vi "Read_Write_Template.vi"(0 "Template File":path, 1 "Mode":T1, 5 "Channel names In":string[](array[string]), 7 "Single Value In":string, 9 "2D Info In":string[][](array[string]), 11 "1D Info In":string[](array[string]), 12 "Save file":bool=TRUE, 13 "Data type":string="Tolerance") -> (3 "Freshly Loaded?":bool, 4 "Template File Out":path, 6 "Template Ch Names Out":string[](array[string]), 8 "Single Value Out":string, 10 "2D Info Out":string[][](array[string]), 14 "Template Info":string[][](array[string]), 15 "1D Info Out":string[](array[string]))   [LabVIEW 2015]
uses:
  Controls/Global_mode.ctl
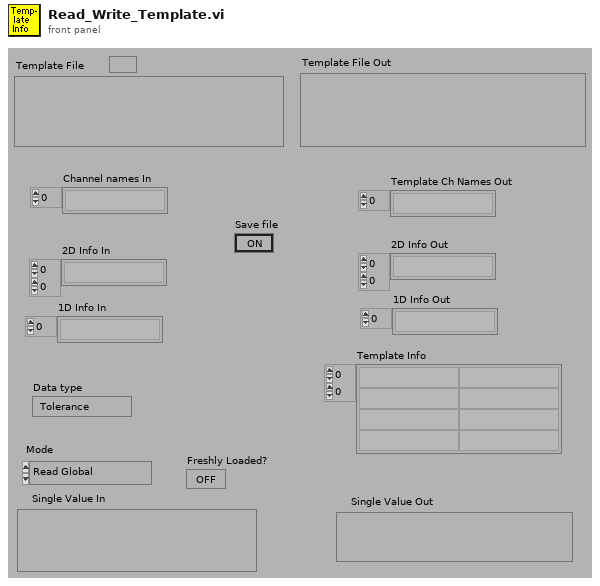
[diagram p1: front panel]
types:
  T1 = typedef "Global_mode.ctl" = enum16{"Read Global", "Load Global From File", "Write Global to File"}
  T2 = typedef "File_Status.ctl" = enum16{"Invalid Path", "This is a folder pathname", "Generic File Error", "Directory structure cannot be created", "File cannot be created", "File can be created", "File exist but read only", "File exist but no access", "File exist with read and write access"}
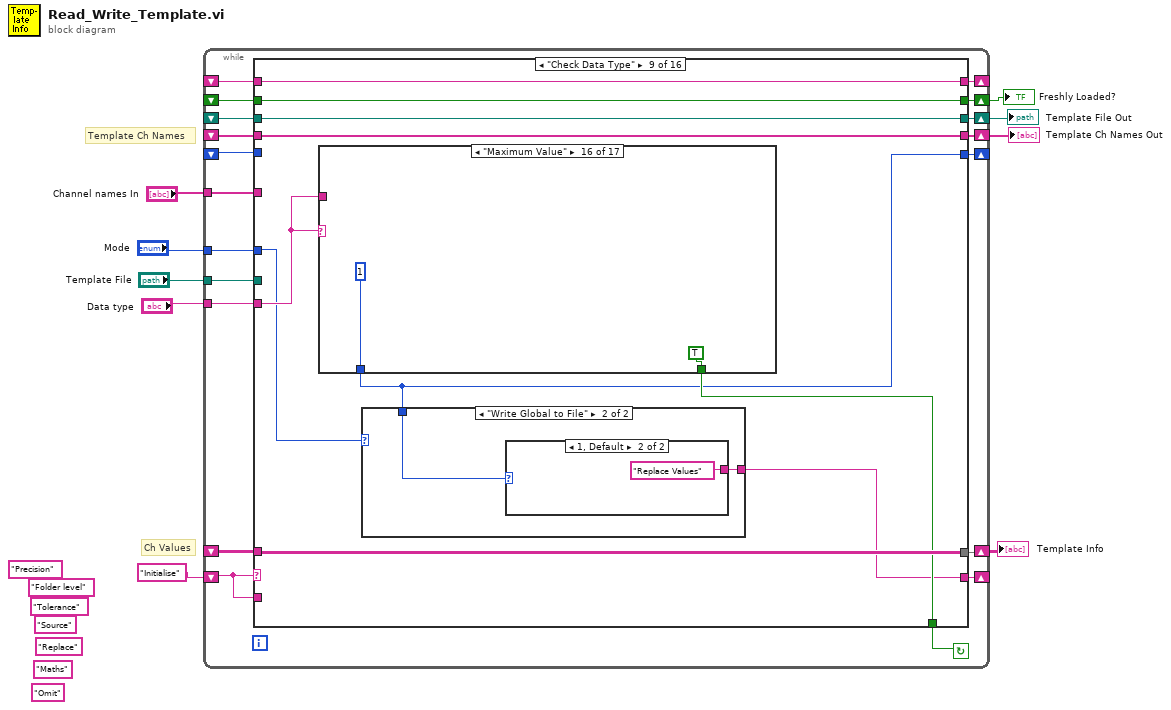
[diagram p0: block diagram]
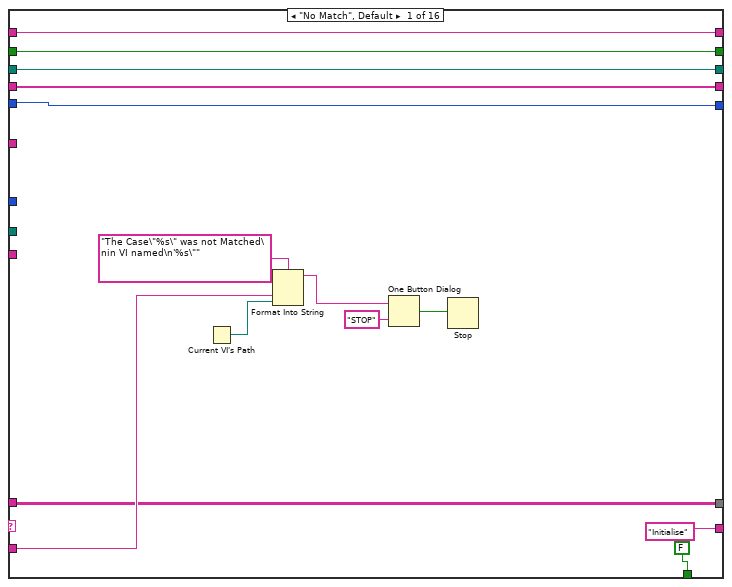
[diagram p2: hidden frame]
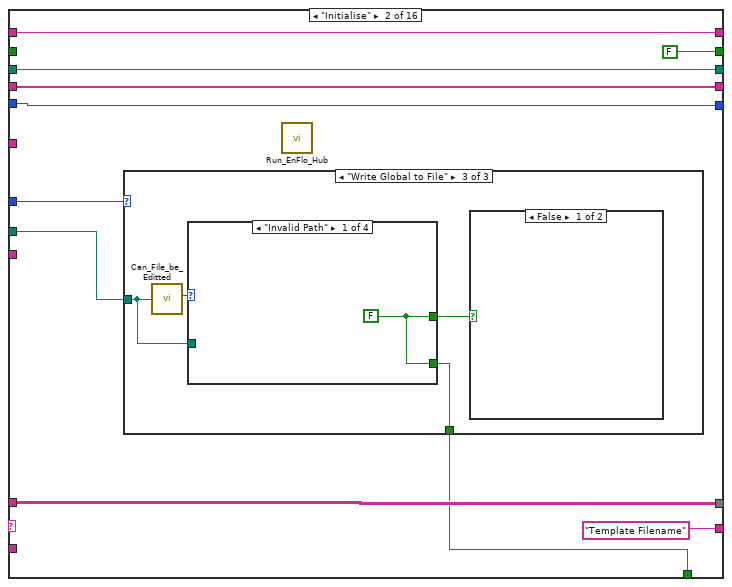
[diagram p3: hidden frame]
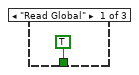
[diagram p4: hidden frame]
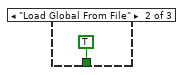
[diagram p5: hidden frame]
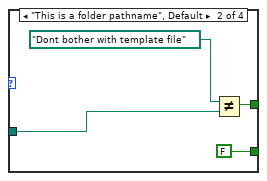
[diagram p6: hidden frame]
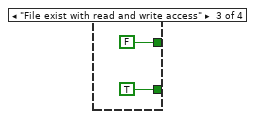
[diagram p7: hidden frame]
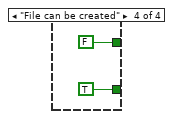
[diagram p8: hidden frame]
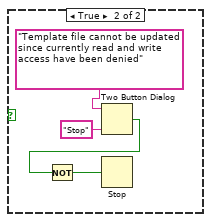
[diagram p9: hidden frame]
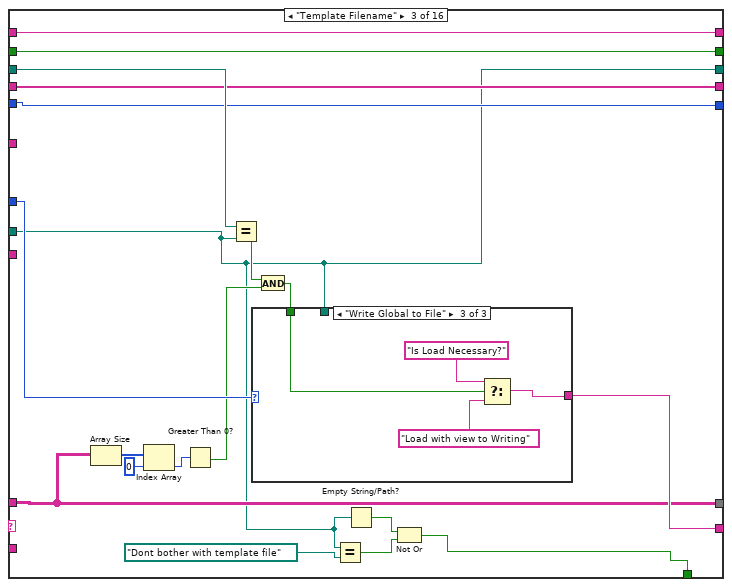
[diagram p10: hidden frame]
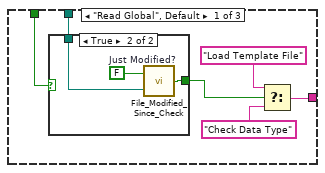
[diagram p11: hidden frame]
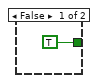
[diagram p12: hidden frame]
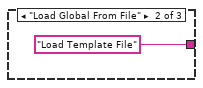
[diagram p13: hidden frame]
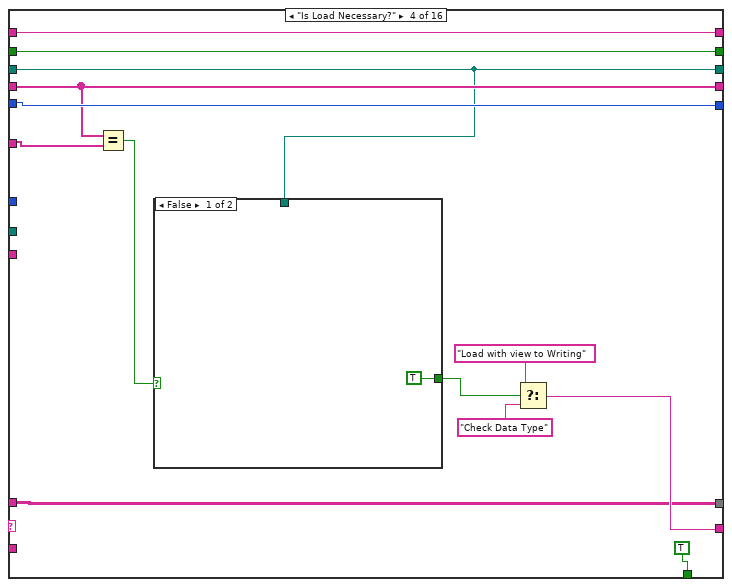
[diagram p14: hidden frame]
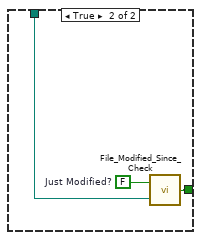
[diagram p15: hidden frame]
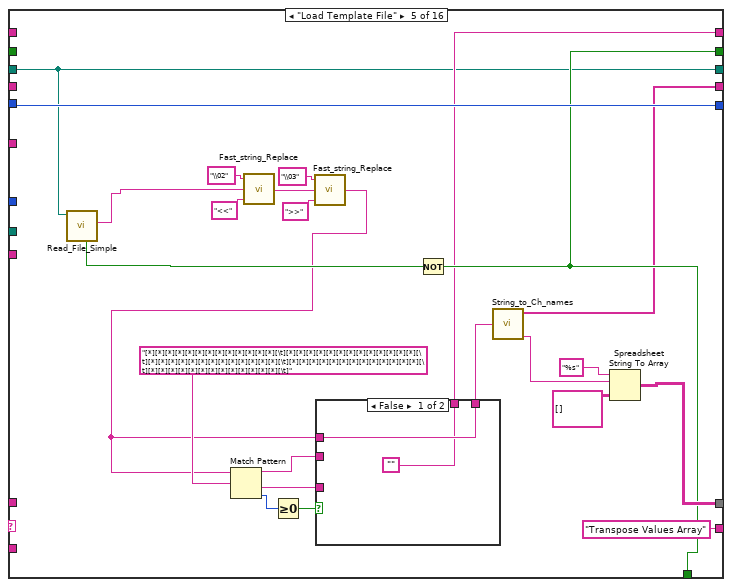
[diagram p16: hidden frame]
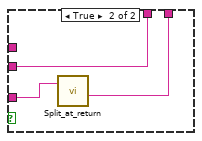
[diagram p17: hidden frame]
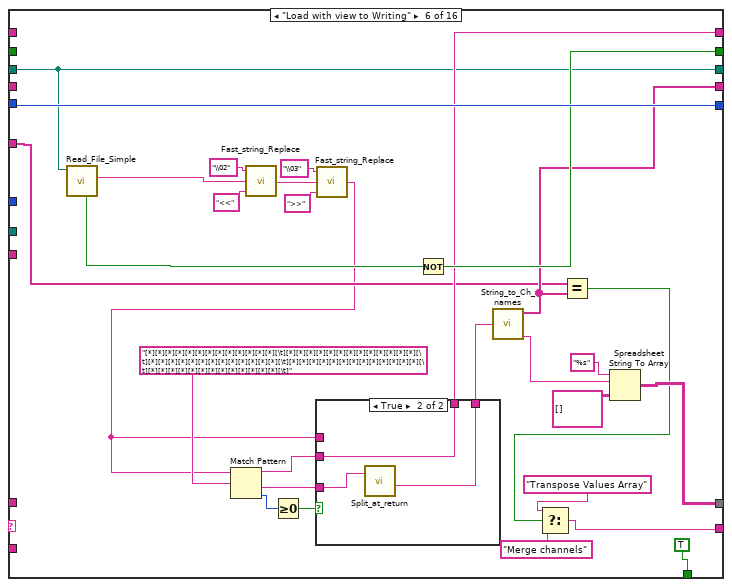
[diagram p18: hidden frame]
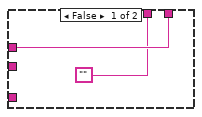
[diagram p19: hidden frame]
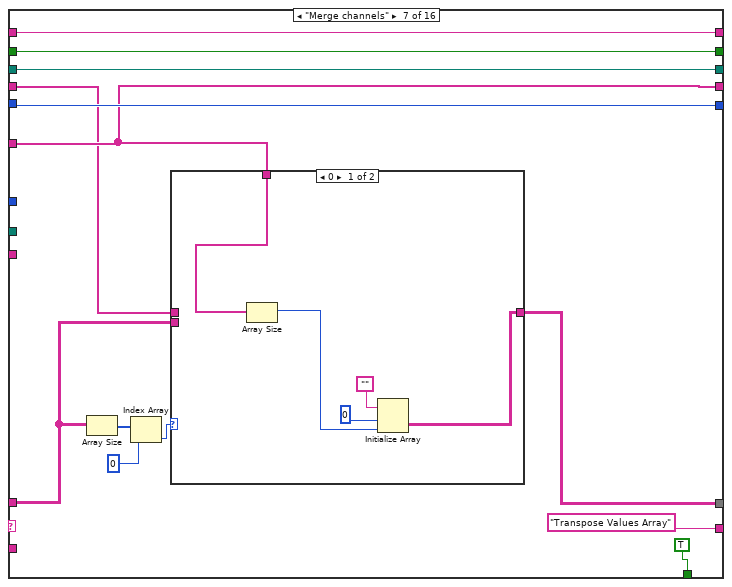
[diagram p20: hidden frame]
diagram:
  (unwired) "Precision"
  (unwired) "Folder level"
  (unwired) "Omit"
  (unwired) "Maths"
  (unwired) "Tolerance"
  (unwired) "Source"
  (unwired) "Replace"
  # "Template Ch Names"
  # "Ch Values"
  n1 = while {
    shift-left: _ -> [w13]
    shift-right: [w14] -> w2
    tunnel: "Channel names In" -> [w16]
    shift-left: _ -> [w15]
    shift-right: [w17] -> _
    tunnel: "Data type" -> [w18]
    shift-left: _ -> [w19]
    shift-right: [w20] -> w5
    shift-left: _ -> [w23]
    shift-right: [w22] -> w6
    shift-left: _ -> [w24]
    shift-right: [w25] -> w7
    tunnel: "Mode" -> [w26]
    shift-left: "Initialise" -> [w21]
    shift-right: [w27] -> _
    shift-right: [w12] -> _
    shift-left: _ -> [w11]
    tunnel: "Template File" -> [w10]
    stop <- w28 continue-if-true
    n2 = case shown="\"Check Data Type\"" w21 {
      tunnel: [FALSE w43 w73 TRUE w139 TRUE ("Save file") TRUE ("Save file") TRUE w231 FALSE FALSE FALSE "Save file" FALSE ("Save file") w461 FALSE] -> w28
      tunnel: ["Initialise" "Template Filename" w87 w118 "Transpose Values Array" w162 "Transpose Values Array" "Check Data Type" w228 "" "" "" "Save Template File" "End" w458 "End"] -> w27
      tunnel: w26 -> [_ w45 w88 _ _ _ _ _ w230 _ _ _ _ _ _ _]
      tunnel: [w33 w51 w83 w112 w143 w178 w191 w218 w234 w300 w314 w334 w360 w447 w456 w506] -> w25
      tunnel: w24 -> [w33 w51 w83 w112 _ _ w189 w217 w234 w300 w314 w334 w361 w447 w455 w506]
      tunnel: w23 -> [w35 w52 w90 w108 w131 w159 w194 w213 w233 w302 w320 w336 w362 w441 w460 w505]
      tunnel: [w35 w52 w72 w108 w131 w159 w194 w213 w233 w302 w320 w336 w362 w441 w460 w505] -> w22
      tunnel: w21 -> [w37 _ _ _ _ _ _ _ _ _ _ _ _ _ _ _]
      tunnel: [w36 w50 w89 w111 w130 w166 w193 w212 w232 w298 w315 w331 w355 w450 w459 w504] -> w20
      tunnel: w19 -> [w36 w50 w89 w111 _ _ w192 w212 w232 w298 w315 w331 w355 w450 w459 w504]
      tunnel: w18 -> [_ _ _ _ _ _ _ _ w235 w301 w312 w335 w358 w443 _ _]
      tunnel: [w31 w48 w82 w116 w145 w180 w197 w211 w229 w291 w317 w323 w353 w449 w457 w502] -> w17
      tunnel: w16 -> [_ _ _ w110 _ w165 w193 _ _ w292 _ w328 w354 _ _ _]
      tunnel: w15 -> [w31 w48 w82 w116 w145 w180 w197 w211 _ w291 w317 w323 w353 w449 w457 w502]
      tunnel: [w30 FALSE w78 w107 w139 w174 w195 w209 w227 w290 w316 w322 w352 w448 w454 w500] -> w14
      tunnel: w13 -> [w30 _ w78 w107 _ _ w195 w209 w227 w290 w316 w322 w352 w448 w454 w500]
      tunnel: [w29 w46 w77 w106 w133 w168 w196 w208 w226 w289 w313 w321 w350 w445 w452 w499] -> w12
      tunnel: w11 -> [w29 w46 w77 w106 _ _ w196 w208 w226 w289 w313 w321 w350 w444 w453 w499]
      tunnel: w10 -> [_ w44 w72 _ _ _ _ _ _ _ _ _ _ _ _ _]
      frame "No Match", Default {
        n3 = Current VI's Path() -> (path=w38:path)
        n4 = Format Into String(format string="The Case\"%s\" was not Matched\nin VI named\n'%s\"" ("Format String"), w37, w38) -> (resulting string=w41:string)  [unwired: 2 in, 1 out]
        n5 = One Button Dialog(message=w41, button name ("OK")="STOP") -> (true=w39:bool)
        n6 = Stop(stop? (T)=w39) -> ()
      }
      frame "Initialise" {
        n7 = case shown="\"Write Global to File\"" w45 {
          tunnel: w44 -> [_ _ w55]
          tunnel: [TRUE TRUE w56] -> w43
          frame "Read Global" {
          }
          frame "Load Global From File" {
          }
          frame "Write Global to File" {
            n8 = call "Can_File_be_Editted.vi"("Filename"=w55) -> ("File Status"=w58:T2)  [unwired: 3 out]
            n9 = case shown="\"Invalid Path\"" w58 {
              tunnel: [w59 w61 FALSE FALSE] -> w57
              tunnel: [w59 FALSE TRUE TRUE] -> w56
              tunnel: w55 -> [_ w60 _ _]
              frame "Invalid Path" {
                w59 = FALSE
              }
              frame "This is a folder pathname", Default {
                n10 = Not Equal?(x=path "Dont bother with template file" ("Template File"), y=w60) -> (x != y?=w61:bool)
              }
              frame "File exist with read and write access" {
              }
              frame "File can be created" {
              }
            }
            n11 = case shown="False" w57 {
              frame False {
              }
              frame True {
                n12 = Two Button Dialog(message="Template file cannot be updated since currently read and write access have been denied", 1:"Stop" ("F button name (\"Cancel\")")) -> (T button?=w69:bool)  [unwired: 1 out]
                n13 = Not(x=w69) -> (.not. x?=w68:bool)
                n14 = Stop(stop? (T)=w68) -> ()
              }
            }
          }
        }
        n15 = call "Run_EnFlo_Hub.vi"() -> ()  [unwired: 8 out]
      }
      frame "Template Filename" {
        n16 = Array Size(array=w83) -> (size(s)=w84:i32[])
        n17 = Index Array(array=w84, index=0 ("Index")) -> (element=w86:i32)
        n18 = Greater Than 0?(x=w86) -> (x > 0?=w79:bool)
        n19 = Equal?(x=w90, y=w72) -> (x = y?=w81:bool)
        n20 = And(x=w81, y=w79) -> (x .and. y?=w80:bool)
        n21 = case shown="\"Write Global to File\"" w88 {
          tunnel: w80 -> [w96 _ w105]
          tunnel: [w92 "Load Template File" w103] -> w87
          tunnel: w72 -> [w95 _ _]
          frame "Read Global", Default {
            n22 = case shown="True" w96 {
              tunnel: w95 -> [_ w100]
              tunnel: [TRUE ("Modified?") w99] -> w94
              frame False {
              }
              frame True {
                w98 = FALSE  # Just Modified?
                n23 = call "File_Modified_Since_Check.vi"("Pathname"=w100, "Just Modified?"=w98) -> ("Modified?"=w99:bool)
              }
            }
            n24 = Select(t="Load Template File", s=w94, f="Check Data Type") -> (s? t:f=w92:string)
          }
          frame "Load Global From File" {
          }
          frame "Write Global to File" {
            n25 = Select(t="Is Load Necessary?", s=w105, f="Load with view to Writing") -> (s? t:f=w103:string)
          }
        }
        n26 = Equal?(x=w72, y=path "Dont bother with template file" ("Template File")) -> (x = y?=w75:bool)
        n27 = Empty String/Path?(string/path=w72) -> (empty?=w74:bool)
        n28 = Not Or(1:w75, 2:w74) -> (0:w73:bool)
      }
      frame "Is Load Necessary?" {
        n29 = Equal?(x=w111, y=w110) -> (x = y?=w109:bool)
        n30 = case shown="False" w109 {
          tunnel: w108 -> [_ w122]
          tunnel: [TRUE ("Modified?") w121] -> w115
          frame False {
          }
          frame True {
            w120 = FALSE  # Just Modified?
            n31 = call "File_Modified_Since_Check.vi"("Pathname"=w122, "Just Modified?"=w120) -> ("Modified?"=w121:bool)
          }
        }
        n32 = Select(t="Load with view to Writing", s=w115, f="Check Data Type") -> (s? t:f=w118:string)
      }
      frame "Load Template File" {
        n33 = call "Read_File_Simple.vi"("Filename"=w131) -> ("Error?"=w144:bool, "string"=w129:string)  [unwired: 2 in, 6 out]
        n34 = call "Fast_string_Replace.vi"("Replace match with:"="<<" ("regular expression"), "Input String"=w129, "regular expression"="\\02") -> ("Output String"=w123:string)  [unwired: 2 out]
        n35 = call "Fast_string_Replace.vi"("Replace match with:"=">>" ("regular expression"), "Input String"=w123, "regular expression"="\\03") -> ("Output String"=w128:string)  [unwired: 2 out]
        n36 = Match Pattern(string=w128, regular expression="[*][*][*][*][*][*][*][*][*][*][*][*][*][\t][*][*][*][*][*][*][*][*][*][*][*][*][*][\t][*][*][*][*][*][*][*][*][*][*][*][*][*][\t][*][*][*][*][*][*][*][*][*][*][*][*][*][\t][*][*][*][*][*][*][*][*][*][*][*][*][*][\t]" ("String")) -> (before substring=w132:string, after substring=w137:string, offset past match=w136:i32)  [unwired: 2 out]
        n37 = Greater Or Equal To 0?(x=w136) -> (x >= 0?=w135:bool)
        n38 = case shown="False" w135 {
          tunnel: w137 -> [_ w151]
          tunnel: [w148 w150] -> w134
          tunnel: w128 -> [w148 _]
          tunnel: ["" w149] -> w133
          tunnel: w132 -> [_ w149]
          frame False {
          }
          frame True {
            n39 = call "Split_at_return.vi"("String"=w151) -> ("after substring"=w150:string)  [unwired: 1 in, 3 out]
          }
        }
        n40 = Not(x=w144) -> (.not. x?=w139:bool)
        n41 = call "String_to_Ch_names.vi"("Spreadsheet string"=w134) -> ("Ch names"=w130:string[], "String After names"=w140:string)  [unwired: 2 out]
        n42 = Spreadsheet String To Array(format string="%s", spreadsheet string=w140, array type (2D Dbl)=string[][] [] ("Channel Values")) -> (array=w143:string[][])  [unwired: 1 out]
      }
      frame "Load with view to Writing" {
        n43 = call "Read_File_Simple.vi"("Filename"=w159) -> ("Error?"=w179:bool, "string"=w153:string)  [unwired: 2 in, 6 out]
        n44 = call "Fast_string_Replace.vi"("Replace match with:"="<<" ("regular expression"), "Input String"=w153, "regular expression"="\\02") -> ("Output String"=w154:string)  [unwired: 2 out]
        n45 = call "Fast_string_Replace.vi"("Replace match with:"=">>" ("regular expression"), "Input String"=w154, "regular expression"="\\03") -> ("Output String"=w152:string)  [unwired: 2 out]
        n46 = Match Pattern(string=w152, regular expression="[*][*][*][*][*][*][*][*][*][*][*][*][*][\t][*][*][*][*][*][*][*][*][*][*][*][*][*][\t][*][*][*][*][*][*][*][*][*][*][*][*][*][\t][*][*][*][*][*][*][*][*][*][*][*][*][*][\t][*][*][*][*][*][*][*][*][*][*][*][*][*][\t]" ("String")) -> (before substring=w167:string, after substring=w172:string, offset past match=w171:i32)  [unwired: 2 out]
        n47 = Greater Or Equal To 0?(x=w171) -> (x >= 0?=w170:bool)
        n48 = case shown="True" w170 {
          tunnel: w172 -> [_ w185]
          tunnel: [w182 w184] -> w169
          tunnel: w152 -> [w182 _]
          tunnel: ["" w183] -> w168
          tunnel: w167 -> [_ w183]
          frame False {
          }
          frame True {
            n49 = call "Split_at_return.vi"("String"=w185) -> ("after substring"=w184:string)  [unwired: 1 in, 3 out]
          }
        }
        n50 = Not(x=w179) -> (.not. x?=w174:bool)
        n51 = call "String_to_Ch_names.vi"("Spreadsheet string"=w169) -> ("Ch names"=w166:string[], "String After names"=w175:string)  [unwired: 2 out]
        n52 = Equal?(x=w165, y=w166) -> (x = y?=w164:bool)
        n53 = Select(t="Transpose Values Array", s=w164, f="Merge channels") -> (s? t:f=w162:string)
        n54 = Spreadsheet String To Array(format string="%s", spreadsheet string=w175, array type (2D Dbl)=string[][] [] ("Channel Values")) -> (array=w178:string[][])  [unwired: 1 out]
      }
      frame "Merge channels" {
        n55 = Array Size(array=w189) -> (size(s)=w188:i32[])
        n56 = Index Array(array=w188, index=0) -> (element=w186:i32)
        n57 = case shown="0" w186 {
          tunnel: w193 -> [w200 w207]
          tunnel: w192 -> [_ w206]
          tunnel: w189 -> [_ w205]
          tunnel: [w199 w204] -> w191
          frame 0 {
            n58 = Array Size(array=w200) -> (size(s)=w201:i32)
            n59 = Initialize Array("", 0 ("Dimension Size"), w201) -> (w199:string[][])
          }
          frame 1, Default {
            n60 = call "Merge_2D_values.vi"("Values In"=w205, "Present Channels"=w206, "Desired Channels"=w207) -> ("Values Out"=w204:string[][])
          }
        }
      }
      frame "Transpose Values Array" {
        n61 = Array Size(array=w217) -> (size(s)=w215:i32[])
        n62 = Index Array(array=w215, index=1 ("Index")) -> (element=w214:i32)
        n63 = for {
          N: w214 -> [_]
          tunnel: w217 -> [w222]
          tunnel: [w223] -> w218 mode=indexing
          i -> [w221]
          n64 = Index Array(array=w222, index (col)=w221) -> (element=w220:string[])  [unwired: 1 in]
          n65 = for {
            tunnel: [w225] -> w223 mode=indexing
            tunnel: w220 -> [w224] mode=indexing
            n66 = call "Remove_Quotes.vi"("String"=w224) -> ("String Out"=w225:string)
          }
        }
      }
      frame "Check Data Type" {
        n67 = case shown="\"Maximum Value\"" w235 {
          tunnel: [1 1 1 1 1 2 1 1 2 2 2 1 2 1 1 1 0] -> w229
          tunnel: w235 -> [w246 _ _ _ _ _ _ _ _ _ _ _ _ _ _ _ _]
          tunnel: [w245 TRUE TRUE TRUE TRUE TRUE TRUE TRUE TRUE TRUE TRUE TRUE TRUE TRUE TRUE TRUE TRUE] -> w231
          frame "No Match", Default {
            n68 = Empty String/Path?(string/path=w246) -> (empty?=w247:bool)
            n69 = case shown="False" w247 {
              tunnel: w246 -> [w250 _]
              tunnel: [FALSE FALSE] -> w245
              frame False {
                n70 = Current VI's Path() -> (path=w251:path)
                n71 = Format Into String(format string="The Case\"%s\" was not Matched\nin VI named\n'%s\"" ("Format String"), w250, w251) -> (resulting string=w254:string)  [unwired: 2 in, 1 out]
                n72 = One Button Dialog(message=w254, button name ("OK")="STOP") -> (true=w252:bool)
                n73 = Stop(stop? (T)=w252) -> ()
              }
              frame True {
              }
            }
          }
          frame "Description" {
          }
          frame "Dispose" {
          }
          frame "Decimal" {
          }
          frame "Precision" {
          }
          frame "Multiple Sources" {
          }
          frame "Summarise" {
          }
          frame "Tolerance" {
          }
          frame "Source" {
          }
          frame "Replace" {
          }
          frame "Ignore When" {
          }
          frame "Maths" {
          }
          frame "Omit" {
          }
          frame "Folder level" {
          }
          frame "Minimum Value" {
          }
          frame "Maximum Value" {
          }
          frame "Log Folder Name" {
          }
        }
        n74 = case shown="\"Write Global to File\"" w230 {
          tunnel: w229 -> [w237 w241]
          tunnel: [w236 w242] -> w228
          frame "Read Global", Default {
            n75 = case shown="0" w237 {
              tunnel: ["Create Outputs 2D" "Create Outputs 1D" "Create single value output"] -> w236
              frame 2, Default {
              }
              frame 1 {
              }
              frame 0 {
              }
            }
          }
          frame "Write Global to File" {
            n76 = case shown="1, Default" w241 {
              tunnel: ["Replace single value" "Replace Values"] -> w242
              frame 0 {
              }
              frame 1, Default {
              }
            }
          }
        }
      }
      frame "Create Outputs 1D" {
        n77 = for {
          tunnel: w301 -> [w310]
          tunnel: w300 -> [w309] mode=indexing
          tunnel: [w308] -> w299 mode=indexing
          n78 = call "Get_Array_Subset.vi"("String Array In"=w309, "Subset Name"=w310) -> ("First Element"=w308:string)  [unwired: 4 out]
        }
        n79 = Array Size(array=w292) -> (size(s)=w294:i32)
        n80 = Equal To 0?(x=w294) -> (x = 0?=w293:bool)
        n81 = case shown="False" w293 {
          tunnel: w299 -> [w306 w307]
          tunnel: w292 -> [w305 _]
          tunnel: w298 -> [w304 _]
          tunnel: [w303 w307] -> w297
          frame False {
            n82 = call "Merge_row_values.vi"("Present Row values"=w306, "Present Channels"=w304, "Desired Channels"=w305) -> ("Desired Row values"=w303:string[])  [unwired: 1 out]
          }
          frame True {
          }
        }
        "1D Info Out" <- w297
      }
      frame "Create single value output" {
        n83 = call "Get_Characters_from_string.vi"("Input string"=w313, "Variable name"=w312) -> ("Value"=→"Single Value Out":string)  [unwired: 1 in, 1 out]
      }
      frame "Create Outputs 2D" {
        n84 = for {
          tunnel: w335 -> [w349]
          tunnel: w334 -> [w348] mode=indexing
          tunnel: [w347] -> w330 mode=indexing
          n85 = call "Get_Array_Subset.vi"("String Array In"=w348, "Subset Name"=w349) -> ("Array Subset Out"=w347:string[])  [unwired: 4 out]
        }
        n86 = Equal?(x=w331, y=w328) -> (x = y?=w326:bool)
        n87 = Array Size(array=w328) -> (size(s)=w327:i32)
        n88 = Equal To 0?(x=w327) -> (x = 0?=w325:bool)
        n89 = Or(x=w326, y=w325) -> (x .or. y?=w324:bool)
        n90 = case shown="False" w324 {
          tunnel: w331 -> [w340 _]
          tunnel: w328 -> [w339 _]
          tunnel: w330 -> [w338 w346]
          tunnel: [w337 w346] -> w329
          frame False {
            n91 = for {
              tunnel: w340 -> [w345]
              tunnel: w339 -> [w344] mode=indexing
              tunnel: w338 -> [w342]
              tunnel: [w341] -> w337 mode=indexing
              n92 = Search 1D Array(1D array=w345, element=w344) -> (index of element=w343:i32)  [unwired: 1 out]
              n93 = Index Array(array=w342, index (row)=w343) -> (element=w341:string[])  [unwired: 1 in]
            }
          }
          frame True {
          }
        }
        "2D Info Out" <- w329
      }
      frame "Replace Values" {
        n94 = for {
          tunnel: w358 -> [w371]
          tunnel: w361 -> [w370] mode=indexing
          tunnel: [w369] -> w360 mode=indexing
          tunnel: w355 -> [w368] mode=indexing
          tunnel: w353 -> [w367]
          tunnel: "1D Info In" -> [w366]
          tunnel: "2D Info In" -> [w365]
          tunnel: w355 -> [w364] mode=indexing
          tunnel: w354 -> [w363]
          n95 = stacked-sequence {
            seq-local: [_ w381 _ _ _] -> [_ _ _ w432 _]
            seq-local: [_ w380 _ _ _] -> [_ _ _ w433 _]
            seq-local: [_ _ w392 _ _] -> [_ _ _ w431 _]
            seq-local: [_ w379 _ _ _] -> [_ _ w388 _ _]
            seq-local: [w374 _ _ _ _] -> [_ _ w389 _ _]
            seq-local: [w372 _ _ _ _] -> [_ _ w387 _ _]
            tunnel: w371 -> [_ w386 _ w434 _]
            tunnel: w370 -> [_ w383 _ _ _]
            tunnel: [_ _ _ w424 _] -> w369
            tunnel: w368 -> [_ _ _ w425 _]
            tunnel: w367 -> [w373 _ _ _ _]
            tunnel: w366 -> [_ _ w391 _ _]
            tunnel: w365 -> [_ _ w390 _ _]
            tunnel: w364 -> [w376 _ _ _ _]
            tunnel: w363 -> [w375 _ _ _ _]
            frame #0 {
              n96 = Search 1D Array(1D array=w375, element=w376) -> (index of element=w372:i32)  [unwired: 1 out]
              n97 = case shown="0, Default" w372 {
                tunnel: [w377 0] -> w374
                tunnel: w373 -> [w377 _]
                frame 0, Default {
                }
                frame -1 {
                }
              }
            }
            frame #1 {
              n98 = call "Get_Array_Subset.vi"("String Array In"=w383, "Subset Name"=w386) -> ("index after match"=w382:i32, "Array Subset Out"=w379:string[], "Length before match"=w384:i32)  [unwired: 2 out]
              n99 = Array Subset(array=w383, index=0 ("Array Index"), length=w384) -> (w381:string[])
              n100 = Array Subset(array=w383, index=w382) -> (w380:string[])  [unwired: 1 in]
            }
            frame #2 {
              n101 = case shown="2, Default" w389 {
                tunnel: [w396 w420 w423] -> w392
                tunnel: w391 -> [_ w422 _]
                tunnel: w390 -> [w395 _ _]
                tunnel: w388 -> [_ _ w423]
                tunnel: w387 -> [w393 w419 _]
                frame 2, Default {
                  n102 = Index Array(array=w395, index (row)=w393) -> (element=w394:string[])  [unwired: 1 in]
                  n103 = while {
                    shift-left: _ -> [w397]
                    shift-right: [w398] -> _
                    tunnel: [w399] -> w396
                    tunnel: w394 -> [w401]
                    i -> [w402]
                    stop <- w400 continue-if-true
                    n104 = case shown="0, Default" w402 {
                      tunnel: w401 -> [w404 w407]
                      tunnel: [w405 FALSE] -> w400
                      tunnel: [w404 w410] -> w399
                      tunnel: [w403 w409] -> w398
                      tunnel: w397 -> [_ w409]
                      frame 0, Default {
                        n105 = Empty String/Path?(string/path=w404) -> (empty?=w403:bool[])
                        n106 = Or Array Elements(Boolean array=w403) -> (logical OR=w405:bool)
                      }
                      frame 1 {
                        n107 = for {
                          shift-right: [w413] -> w410
                          shift-left: string[] [] -> [w412]
                          tunnel: w409 -> [w414] mode=indexing
                          tunnel: w407 -> [w411] mode=indexing
                          n108 = case shown="True" w414 {
                            tunnel: [w416 w418] -> w413
                            tunnel: w412 -> [w417 w418]
                            tunnel: w411 -> [w415 _]
                            frame False {
                              n109 = Build Array (concatenate)(w417, w415) -> (w416:string[])
                            }
                            frame True {
                            }
                          }
                        }
                      }
                    }
                  }
                }
                frame 1 {
                  n110 = Index Array(array=w422, index=w419) -> (element=w421:string)
                  n111 = Build Array(w421) -> (w420:string[])
                }
                frame 0 {
                }
              }
            }
            frame #3 {
              w426 = ""
              n112 = Format Into String(format string="**%s Start**" ("Format String"), w434) -> (resulting string=w430:string)  [unwired: 2 in, 1 out]
              n113 = Format Into String(format string="**%s End**" ("Format String"), w434) -> (resulting string=w429:string)  [unwired: 2 in, 1 out]
              n114 = Build Array (concatenate)(w432, w430, w431, w429, w433) -> (w428:string[])
              n115 = call "Clean_Up_Template.vi"("Template Info In"=w428) -> ("Template Info Out"=w427:string[])
              n116 = Build Array (concatenate)(w426, w425, w426, w427) -> (w424:string[])
            }
            frame #4 {
            }
          }
        }
      }
      frame "Replace single value" {
        w438 = FALSE  # append to file? (new file:F)
        w439 = FALSE  # advisory dialog? (display:T)
        n117 = call "Read_File_Simple.vi"("Filename"=w441) -> ("string"=w442:string)  [unwired: 2 in, 7 out]
        n118 = call "Replace_data_in_setup_string.vi"("New data string"="Single Value In", "Input string"=w444, "Variable name"=w443) -> ("Appended string"=w445:string)
        n119 = call "Replace_data_in_setup_string.vi"("New data string"="Single Value In", "Input string"=w442, "Variable name"=w443) -> ("Appended string"=w440:string)
        n120 = call "Write_Characters_To_File.vi"("file path (dialog if empty)"=w441, "advisory dialog? (display:T)"=w439, "character string"=w440, "append to file? (new file:F)"=w438) -> ()  [unwired: 1 in, 4 out]
      }
      frame "Save Template File" {
        n121 = stacked-sequence {
          seq-local: [w464 _] -> [_ w478]
          tunnel: [_ TRUE] -> w461
          tunnel: w460 -> [_ w488]
          tunnel: w459 -> [_ w487]
          tunnel: [_ "Update last Modified VI"] -> w458
          tunnel: [_ w481] -> w456
          tunnel: w455 -> [_ w480]
          tunnel: w453 -> [w463 _]
          tunnel: [w462 _] -> w452
          frame #0 {
            w469 = "Log Folder Name" ("Variable name")
            n122 = call "Get_Characters_from_string.vi"("Input string"=w463, "Variable name"=w469) -> ("Status"=w470:enum16{"Char in string", "Char not in string"})  [unwired: 1 in, 1 out]
            n123 = case shown="\"Char not in string\"" w470 {
              tunnel: w469 -> [_ w477]
              tunnel: w463 -> [w471 w473]
              tunnel: [w471 w472] -> w462
              frame "Char in string" {
              }
              frame "Char not in string" {
                n124 = Default Directory() -> (w476:path)
                n125 = Path To String(path=w476) -> (string=w475:string)
                n126 = call "Characters_to_string.vi"("Characters to write"=w475, "Label for characters"=w477) -> ("Output string"=w474:string)
                n127 = Concatenate Strings(w473, w474) -> (w472:string)
              }
            }
            n128 = Initialize Array("", 10 ("Dimension Size")) -> (w468:string[])
            n129 = call "Asterisk_header.vi"("Channel names"=w468) -> ("Header string"=w465:string)
            n130 = Concatenate Strings(w462, w465) -> (w464:string)
          }
          frame #1 {
            w486 = FALSE  # exists?
            n131 = Transpose 2D Array(2D array=w480) -> (transposed array=w484:string[][])
            n132 = for {
              shift-right: [w491] -> w482
              shift-left: string[][] [] -> [w490]
              tunnel: w484 -> [w489] mode=indexing
              n133 = Equal?(x=w489, y=" ") -> (x = y?=w493:bool[])
              n134 = And Array Elements(Boolean array=w493) -> (logical AND=w492:bool)
              n135 = case shown="False" w492 {
                tunnel: [w496 w498] -> w491
                tunnel: w490 -> [w497 w498]
                tunnel: w489 -> [w495 _]
                frame False {
                  n136 = Build Array (concatenate)(w497, w495) -> (w496:string[][])
                }
                frame True {
                }
              }
            }
            n137 = Transpose 2D Array(2D array=w482) -> (transposed array=w481:string[][])
            n138 = call "Write_Ch_data_file.vi"("Header string"=w478, "exists?"=w486, "Channel Values"=w482, "Channel names"=w487, "Filename"=w488) -> ()  [unwired: 2 in, 5 out]
          }
        }
      }
      frame "Update last Modified VI" {
        w501 = TRUE  # Just Modified?
        n139 = call "File_Modified_Since_Check.vi"("Pathname"=w505, "Just Modified?"=w501) -> ()  [unwired: 1 out]
      }
    }
  }
  "Template Ch Names Out" <- w5
  "Template File Out" <- w6
  "Template Info" <- w7
  "Freshly Loaded?" <- w2
